vi "IMAQ FPGA CXP Write To Buffer (64 elements).vi"(9 "Reset":bool, 10 "Valid Bytes":u8, 11 "Pixel Data In U8x32":u8[](array[numeric])=[0, 0, 0, 0, 0, 0, 0, 0, 0, 0, 0, 0, 0, 0, 0, 0, 0, 0, 0, 0, 0, 0, 0, 0, 0, 0, 0, 0, 0, 0, 0, 0]) -> (3 "Buffer Out":u8[](array[numeric]))   [LabVIEW 2020]
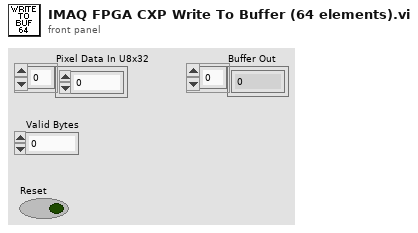
[diagram p1: front panel]
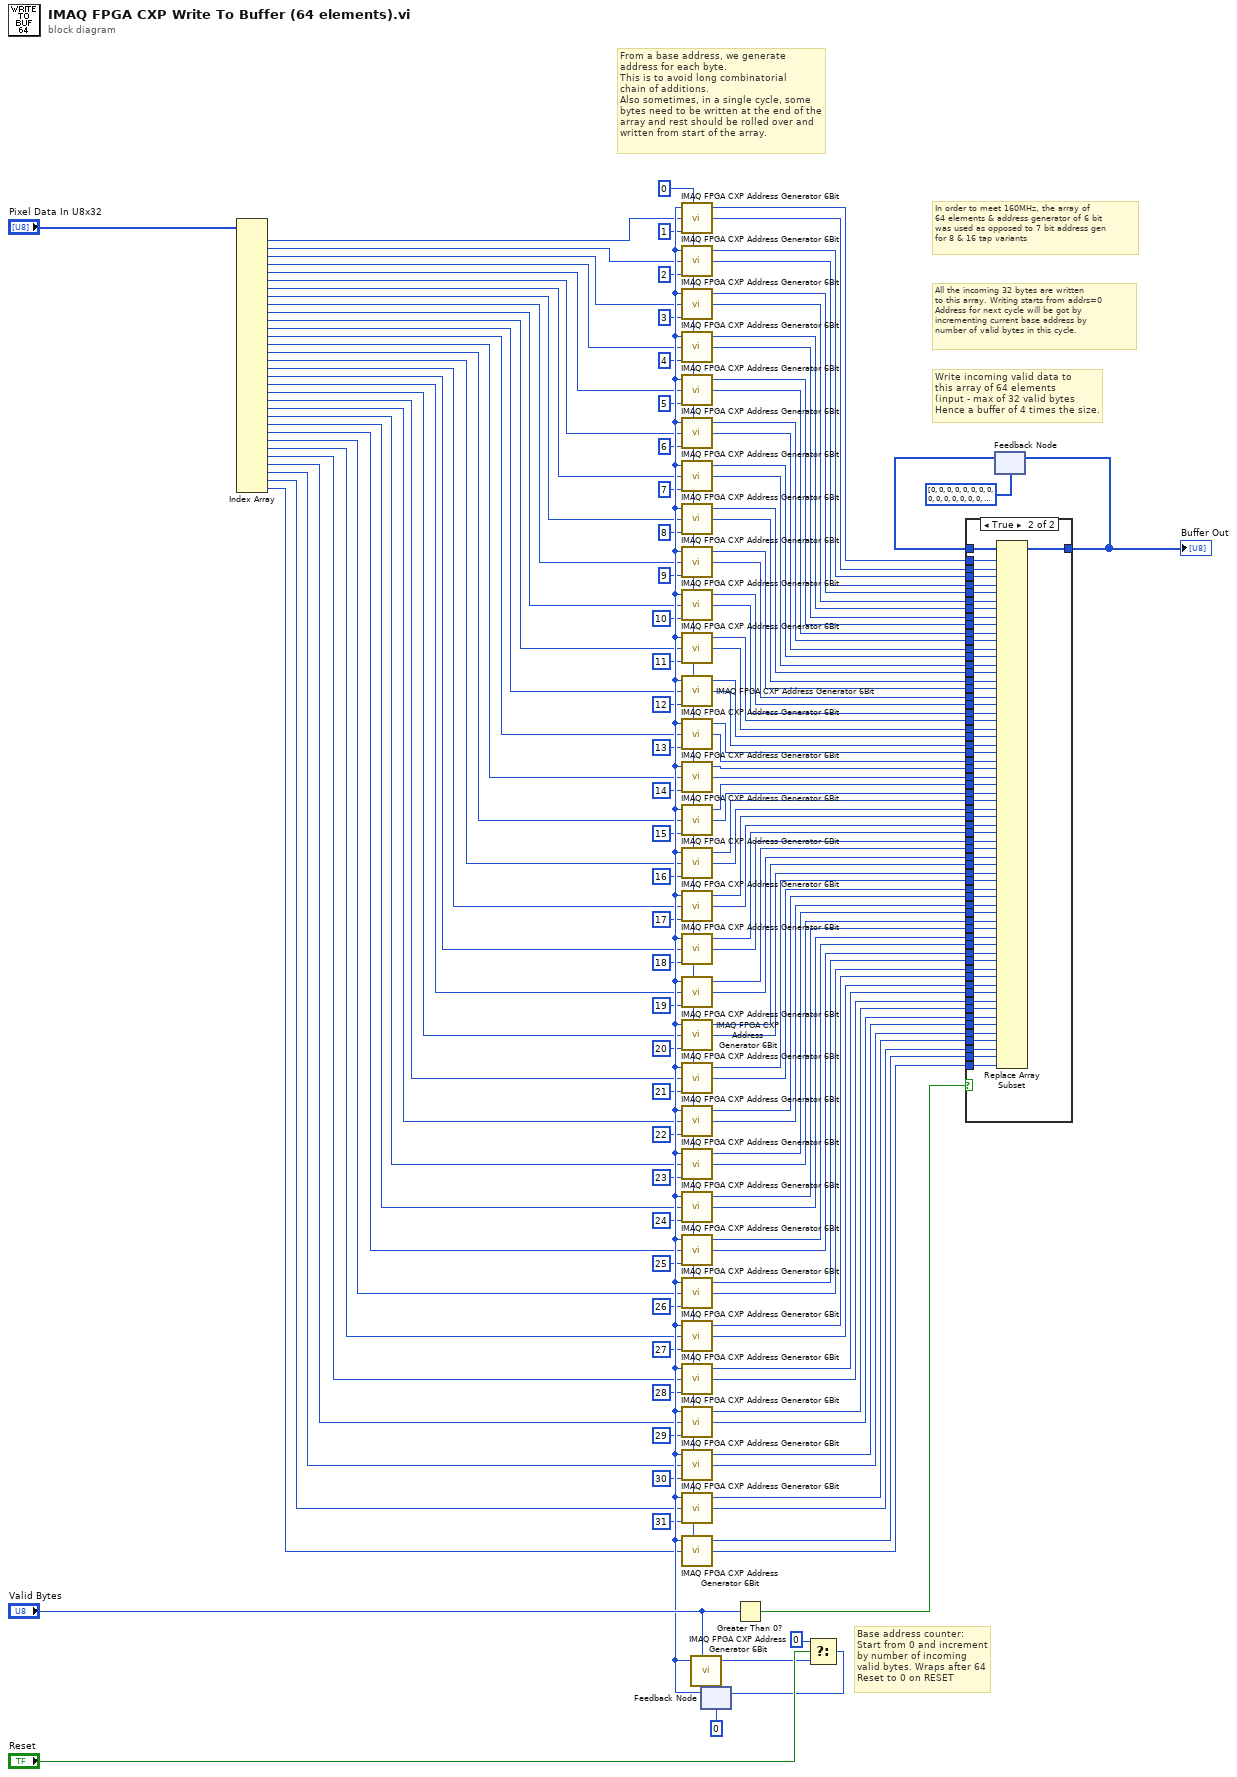
[diagram p0: block diagram]
diagram:
  # "In order to meet 160MHz, the array of\n64 elements & address generator of 6 bit\nwas used as opposed to 7 bit address gen\nfor 8 & 16 tap variants"
  # "Base address counter:\nStart from 0 and increment\nby number of incoming\nvalid bytes. Wraps after 64\nReset to 0 on RESET"
  # "From a base address, we generate\naddress for each byte.\nThis is to avoid long combinatorial\nchain of additions.\nAlso sometimes, in a single cycle, some\nbytes need to be written at the end of the\narray and rest should be rolled over and \nwritten from start of the array."
  # "All the incoming 32 bytes are written\nto this array. Writing starts from addrs=0\nAddress for next cycle will be got by\nincrementing current base address by\nnumber of valid bytes in this cycle."
  # "Write incoming valid data to\nthis array of 64 elements\n(input - max of 32 valid bytes\nHence a buffer of 4 times the size."
  n1 = Index Array(array="Pixel Data In U8x32") -> (element #1=w6:u8, element #2=w7:u8, element #3=w8:u8, element #4=w9:u8, element #5=w10:u8, element #6=w11:u8, element #7=w12:u8, element #8=w13:u8, element #9=w14:u8, element #10=w15:u8, element #11=w16:u8, element #12=w17:u8, element #13=w18:u8, element #14=w19:u8, element #15=w20:u8, element #16=w21:u8, element #17=w22:u8, element #18=w23:u8, element #19=w24:u8, element #20=w25:u8, element #21=w26:u8, element #22=w27:u8, element #23=w28:u8, element #24=w29:u8, element #25=w30:u8, element #26=w31:u8, element #27=w32:u8, element #28=w33:u8, element #29=w34:u8, element #30=w35:u8, element #31=w36:u8, element #32=w37:u8)  [unwired: 32 in]
  n2 = feedback #1(u8 0) -> (w106:u8)
  n3 = call <vilib>:"IMAQ FPGA CXP Address Generator 6Bit.vi"("Base Address"=w106, "Index"=u8 0) -> ("Address Out"=w54:u8)  [unwired: 7 in]
  n4 = call <vilib>:"IMAQ FPGA CXP Address Generator 6Bit.vi"("Base Address"=w106, "Index"=u8 1) -> ("Address Out"=w55:u8)  [unwired: 7 in]
  n5 = call <vilib>:"IMAQ FPGA CXP Address Generator 6Bit.vi"("Base Address"=w106, "Index"=u8 2) -> ("Address Out"=w56:u8)  [unwired: 7 in]
  n6 = call <vilib>:"IMAQ FPGA CXP Address Generator 6Bit.vi"("Base Address"=w106, "Index"=u8 3) -> ("Address Out"=w57:u8)  [unwired: 7 in]
  n7 = call <vilib>:"IMAQ FPGA CXP Address Generator 6Bit.vi"("Base Address"=w106, "Index"=u8 4) -> ("Address Out"=w58:u8)  [unwired: 7 in]
  n8 = call <vilib>:"IMAQ FPGA CXP Address Generator 6Bit.vi"("Base Address"=w106, "Index"=u8 5) -> ("Address Out"=w59:u8)  [unwired: 7 in]
  n9 = call <vilib>:"IMAQ FPGA CXP Address Generator 6Bit.vi"("Base Address"=w106, "Index"=u8 6) -> ("Address Out"=w60:u8)  [unwired: 7 in]
  n10 = call <vilib>:"IMAQ FPGA CXP Address Generator 6Bit.vi"("Base Address"=w106, "Index"=u8 7) -> ("Address Out"=w61:u8)  [unwired: 7 in]
  n11 = call <vilib>:"IMAQ FPGA CXP Address Generator 6Bit.vi"("Base Address"=w106, "Index"=u8 8) -> ("Address Out"=w62:u8)  [unwired: 7 in]
  n12 = call <vilib>:"IMAQ FPGA CXP Address Generator 6Bit.vi"("Base Address"=w106, "Index"=u8 9) -> ("Address Out"=w63:u8)  [unwired: 7 in]
  n13 = call <vilib>:"IMAQ FPGA CXP Address Generator 6Bit.vi"("Base Address"=w106, "Index"=u8 10) -> ("Address Out"=w64:u8)  [unwired: 7 in]
  n14 = call <vilib>:"IMAQ FPGA CXP Address Generator 6Bit.vi"("Base Address"=w106, "Index"=u8 11) -> ("Address Out"=w65:u8)  [unwired: 7 in]
  n15 = call <vilib>:"IMAQ FPGA CXP Address Generator 6Bit.vi"("Base Address"=w106, "Index"=u8 12) -> ("Address Out"=w66:u8)  [unwired: 7 in]
  n16 = call <vilib>:"IMAQ FPGA CXP Address Generator 6Bit.vi"("Base Address"=w106, "Index"=u8 13) -> ("Address Out"=w67:u8)  [unwired: 7 in]
  n17 = call <vilib>:"IMAQ FPGA CXP Address Generator 6Bit.vi"("Base Address"=w106, "Index"=u8 14) -> ("Address Out"=w68:u8)  [unwired: 7 in]
  n18 = call <vilib>:"IMAQ FPGA CXP Address Generator 6Bit.vi"("Base Address"=w106, "Index"=u8 15) -> ("Address Out"=w69:u8)  [unwired: 7 in]
  n19 = call <vilib>:"IMAQ FPGA CXP Address Generator 6Bit.vi"("Base Address"=w106, "Index"=u8 16) -> ("Address Out"=w86:u8)  [unwired: 7 in]
  n20 = call <vilib>:"IMAQ FPGA CXP Address Generator 6Bit.vi"("Base Address"=w106, "Index"=u8 17) -> ("Address Out"=w87:u8)  [unwired: 7 in]
  n21 = call <vilib>:"IMAQ FPGA CXP Address Generator 6Bit.vi"("Base Address"=w106, "Index"=u8 18) -> ("Address Out"=w88:u8)  [unwired: 7 in]
  n22 = call <vilib>:"IMAQ FPGA CXP Address Generator 6Bit.vi"("Base Address"=w106, "Index"=u8 19) -> ("Address Out"=w89:u8)  [unwired: 7 in]
  n23 = call <vilib>:"IMAQ FPGA CXP Address Generator 6Bit.vi"("Base Address"=w106, "Index"=u8 20) -> ("Address Out"=w90:u8)  [unwired: 7 in]
  n24 = call <vilib>:"IMAQ FPGA CXP Address Generator 6Bit.vi"("Base Address"=w106, "Index"=u8 21) -> ("Address Out"=w91:u8)  [unwired: 7 in]
  n25 = call <vilib>:"IMAQ FPGA CXP Address Generator 6Bit.vi"("Base Address"=w106, "Index"=u8 22) -> ("Address Out"=w92:u8)  [unwired: 7 in]
  n26 = call <vilib>:"IMAQ FPGA CXP Address Generator 6Bit.vi"("Base Address"=w106, "Index"=u8 23) -> ("Address Out"=w93:u8)  [unwired: 7 in]
  n27 = call <vilib>:"IMAQ FPGA CXP Address Generator 6Bit.vi"("Base Address"=w106, "Index"=u8 24) -> ("Address Out"=w94:u8)  [unwired: 7 in]
  n28 = call <vilib>:"IMAQ FPGA CXP Address Generator 6Bit.vi"("Base Address"=w106, "Index"=u8 25) -> ("Address Out"=w95:u8)  [unwired: 7 in]
  n29 = call <vilib>:"IMAQ FPGA CXP Address Generator 6Bit.vi"("Base Address"=w106, "Index"=u8 26) -> ("Address Out"=w96:u8)  [unwired: 7 in]
  n30 = call <vilib>:"IMAQ FPGA CXP Address Generator 6Bit.vi"("Base Address"=w106, "Index"=u8 27) -> ("Address Out"=w97:u8)  [unwired: 7 in]
  n31 = call <vilib>:"IMAQ FPGA CXP Address Generator 6Bit.vi"("Base Address"=w106, "Index"=u8 28) -> ("Address Out"=w98:u8)  [unwired: 7 in]
  n32 = call <vilib>:"IMAQ FPGA CXP Address Generator 6Bit.vi"("Base Address"=w106, "Index"=u8 29) -> ("Address Out"=w99:u8)  [unwired: 7 in]
  n33 = call <vilib>:"IMAQ FPGA CXP Address Generator 6Bit.vi"("Base Address"=w106, "Index"=u8 30) -> ("Address Out"=w100:u8)  [unwired: 7 in]
  n34 = call <vilib>:"IMAQ FPGA CXP Address Generator 6Bit.vi"("Base Address"=w106, "Index"=u8 31) -> ("Address Out"=w103:u8)  [unwired: 7 in]
  n35 = call <vilib>:"IMAQ FPGA CXP Address Generator 6Bit.vi"("Base Address"=w106, "Index"="Valid Bytes") -> ("Address Out"=w3:u8)  [unwired: 7 in]
  n36 = Greater Than 0?(x="Valid Bytes") -> (x > 0?=w107:bool)
  n37 = Select(t=u8 0, s="Reset", f=w3) -> (s? t:f=w2:u8)
  n38 = feedback-in #1(w2) -> ()
  n39 = feedback #2(u8[] [0, 0, 0, 0, 0, 0, 0, 0, 0, 0, 0, 0, 0, 0, 0, 0, 0, 0, 0, 0, 0, 0, 0, 0, 0, 0, 0, 0, 0, 0, 0, 0, 0, 0, 0, 0, 0, 0, 0, 0, 0, 0, 0, 0, 0, 0, 0, 0, 0, 0, 0, 0, 0, 0, 0, 0, 0, 0, 0, 0, 0, 0, 0, 0]) -> (w102:u8[])
  n40 = case shown="True" w107 {
    tunnel: w6 -> [_ w175]
    tunnel: w7 -> [_ w174]
    tunnel: w8 -> [_ w173]
    tunnel: w9 -> [_ w172]
    tunnel: w10 -> [_ w171]
    tunnel: w11 -> [_ w170]
    tunnel: w12 -> [_ w169]
    tunnel: w13 -> [_ w168]
    tunnel: w14 -> [_ w167]
    tunnel: w15 -> [_ w166]
    tunnel: w16 -> [_ w165]
    tunnel: w17 -> [_ w164]
    tunnel: w18 -> [_ w163]
    tunnel: w19 -> [_ w162]
    tunnel: w20 -> [_ w161]
    tunnel: w21 -> [_ w160]
    tunnel: w22 -> [_ w159]
    tunnel: w23 -> [_ w158]
    tunnel: w24 -> [_ w157]
    tunnel: w25 -> [_ w156]
    tunnel: w26 -> [_ w155]
    tunnel: w27 -> [_ w154]
    tunnel: w28 -> [_ w153]
    tunnel: w29 -> [_ w152]
    tunnel: w30 -> [_ w151]
    tunnel: w31 -> [_ w150]
    tunnel: w32 -> [_ w149]
    tunnel: w33 -> [_ w148]
    tunnel: w34 -> [_ w147]
    tunnel: w35 -> [_ w146]
    tunnel: w36 -> [_ w145]
    tunnel: w37 -> [_ w144]
    tunnel: w54 -> [_ w143]
    tunnel: w55 -> [_ w142]
    tunnel: w56 -> [_ w141]
    tunnel: w57 -> [_ w140]
    tunnel: w58 -> [_ w139]
    tunnel: w59 -> [_ w138]
    tunnel: w60 -> [_ w137]
    tunnel: w61 -> [_ w136]
    tunnel: w62 -> [_ w135]
    tunnel: w63 -> [_ w134]
    tunnel: w64 -> [_ w133]
    tunnel: w65 -> [_ w132]
    tunnel: w66 -> [_ w131]
    tunnel: w67 -> [_ w130]
    tunnel: w68 -> [_ w129]
    tunnel: w69 -> [_ w128]
    tunnel: w86 -> [_ w127]
    tunnel: w87 -> [_ w126]
    tunnel: w88 -> [_ w125]
    tunnel: w89 -> [_ w124]
    tunnel: w90 -> [_ w123]
    tunnel: w91 -> [_ w122]
    tunnel: w92 -> [_ w121]
    tunnel: w93 -> [_ w120]
    tunnel: w94 -> [_ w119]
    tunnel: w95 -> [_ w118]
    tunnel: w96 -> [_ w117]
    tunnel: w97 -> [_ w116]
    tunnel: w98 -> [_ w115]
    tunnel: w99 -> [_ w114]
    tunnel: w100 -> [_ w113]
    tunnel: w103 -> [_ w112]
    tunnel: w102 -> [w109 w111]
    tunnel: [w109 w110] -> w104
    frame False {
    }
    frame True {
      n41 = Replace Array Subset(array=w111, new element #1=w175, index #1=w143, new element #2=w174, index #2=w142, new element #3=w173, index #3=w141, new element #4=w172, index #4=w140, new element #5=w171, index #5=w139, new element #6=w170, index #6=w138, new element #7=w169, index #7=w137, new element #8=w168, index #8=w136, new element #9=w167, index #9=w135, new element #10=w166, index #10=w134, new element #11=w165, index #11=w133, new element #12=w164, index #12=w132, new element #13=w163, index #13=w131, new element #14=w162, index #14=w130, new element #15=w161, index #15=w129, new element #16=w160, index #16=w128, new element #17=w159, index #17=w127, new element #18=w158, index #18=w126, new element #19=w157, index #19=w125, new element #20=w156, index #20=w124, new element #21=w155, index #21=w123, new element #22=w154, index #22=w122, new element #23=w153, index #23=w121, new element #24=w152, index #24=w120, new element #25=w151, index #25=w119, new element #26=w150, index #26=w118, new element #27=w149, index #27=w117, new element #28=w148, index #28=w116, new element #29=w147, index #29=w115, new element #30=w146, index #30=w114, new element #31=w145, index #31=w113, new element #32=w144, index #32=w112) -> (w110:u8[])
    }
  }
  "Buffer Out" <- w104
  n42 = feedback-in #2(w104) -> ()
